vi "Force Analysis iso.vi"(1 "Dynamic Data Type 2":dynamicdata(waveform)) -> (0 "Dynamic Data Type":dynamicdata(waveform))   [LabVIEW 2016]
uses:
  <vilib>/express/express shared/transition.llb/Dynamic To Waveform Array.vi
  <vilib>/express/express arith-compare/Formula/Block/exnFormulaBlock how many pts in the wave.vi
  <vilib>/express/express shared/ex_Modify Signal Name.vi
  <vilib>/express/express shared/transition.llb/Waveform Array To Dynamic.vi
  <vilib>/express/express arith-compare/Formula/XNode/ExpressFormulaBlockNode.xnode
panel:
  in  "Tab Control":enum32{"Trial A"}(tab)
  out "RFD (PF)":dbl
  out "T to PF (ms)":dbl
  out "Min. Force":dbl
  out "Mean Force":dbl
  out "Impulse-250":dbl
  out "Impulse-200":dbl
  out "Impulse-150":dbl
  out "Impulse-100":dbl
  out "Impulse-PF":dbl
  out "F200":dbl
  out "RFD (250ms)":dbl
  out "RFD (150ms)":dbl
  out "RFD (100ms)":dbl
  out "F250":dbl
  out "F150":dbl
  out "F100":dbl
  out "RFD (200ms)":dbl
  out "PF":dbl
  out "Trial A":dynamicdata(graph) caption="Filtered Signal"
  out "PRFD (5ms)":dbl
  out "PRFD (10ms)":dbl
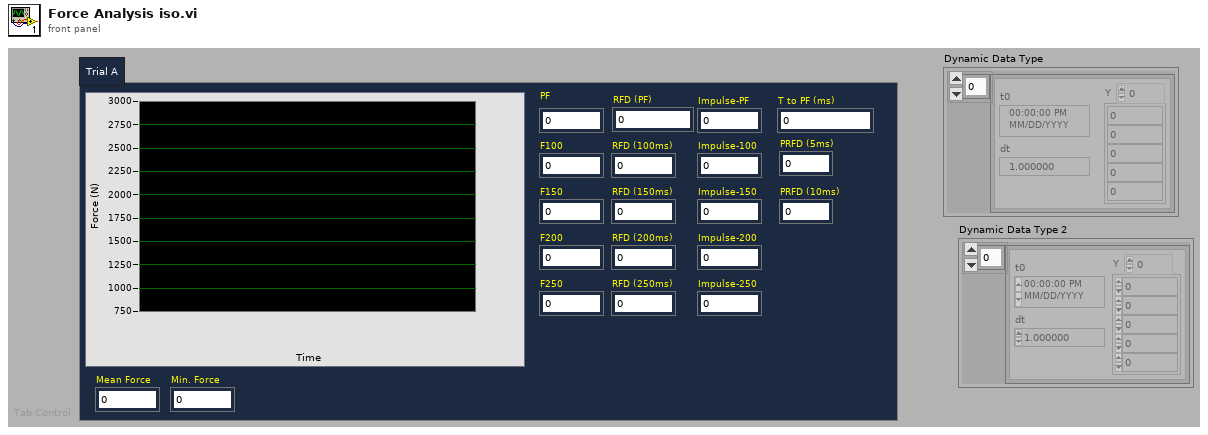
[diagram p1: front panel]
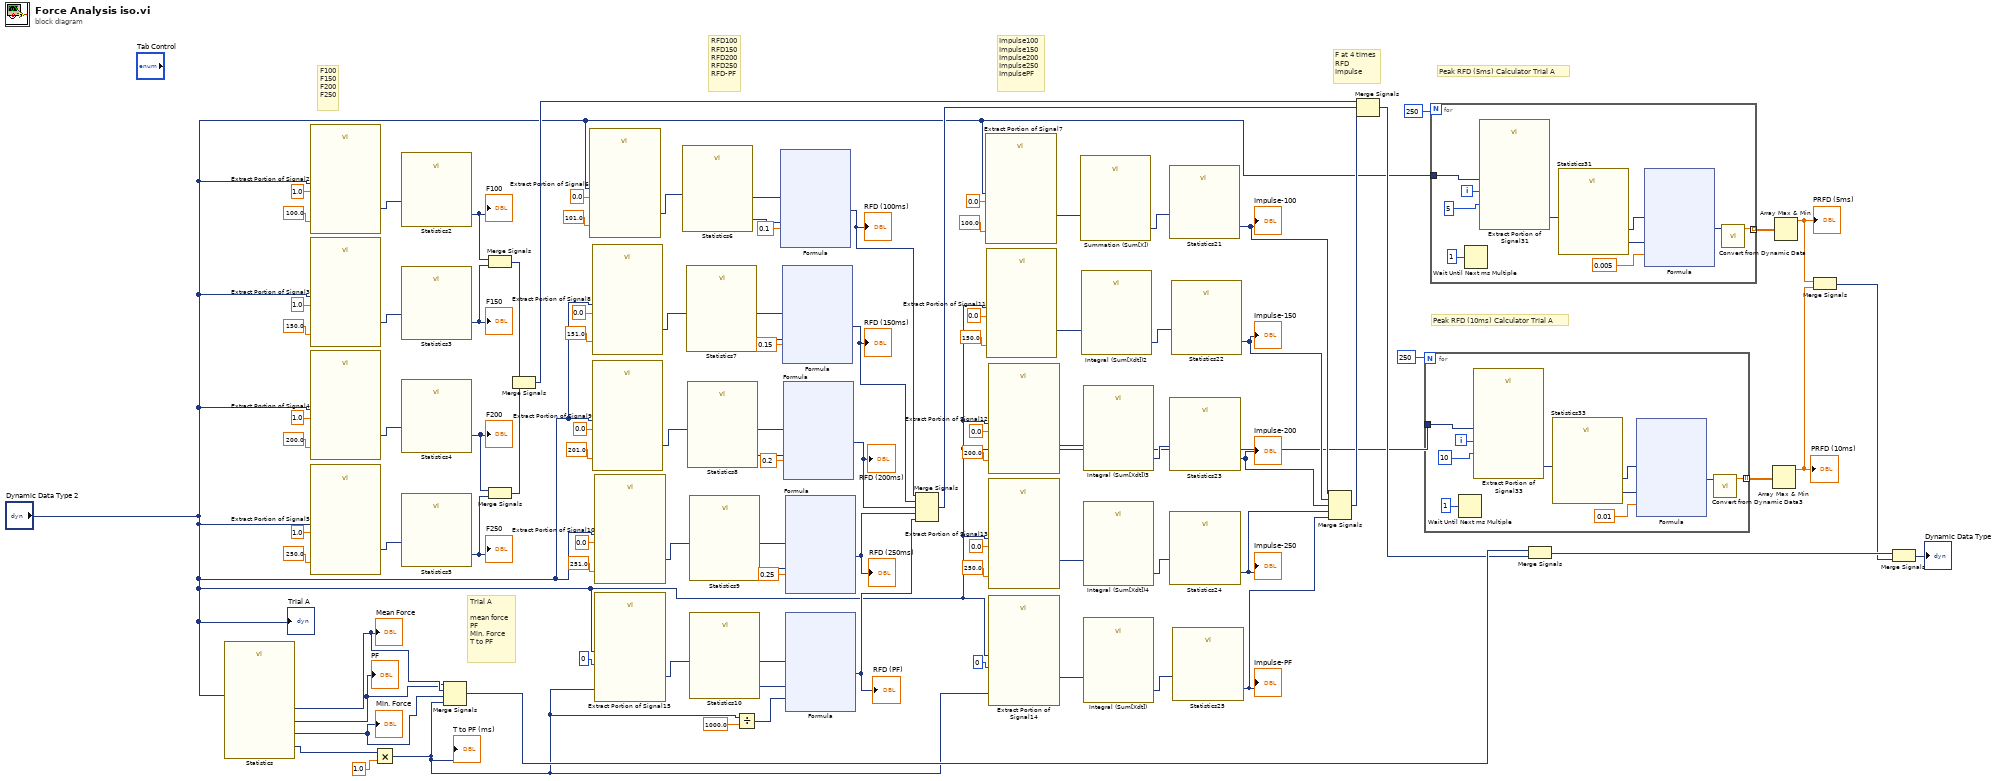
[diagram p0: block diagram]
diagram:
  # "Peak RFD (10ms) Calculator Trial A"
  # "Peak RFD (5ms) Calculator Trial A"
  # "F at 4 times\nRFD\nImpulse"
  # "Impulse100\nImpulse150\nImpulse200\nImpulse250\nImpulsePF"
  # "RFD100\nRFD150\nRFD200\nRFD250\nRFD-PF"
  # "Trial A\n\nmean force\nPF\nMin. Force\nT to PF"
  # "F100\nF150\nF200\nF250"
  n1 = call "Statistics"("Signals"="Dynamic Data Type 2") -> ("Index of Max"=w3:dynamicdata, "Arithmetic Mean"=w2:dynamicdata, "Minimum"=w16:dynamicdata, "Maximum"=w1:dynamicdata)  [unwired: 2 in, 21 out]
  "PF" <- w1
  "Mean Force" <- w2
  "Min. Force" <- w16
  n2 = call "Extract Portion of Signal2"("Samples"=100.0 ("y"), "Begin Sample"=1.0 ("y"), "Signals"="Dynamic Data Type 2") -> ("Section"=w95:dynamicdata)  [unwired: 1 in, 7 out]
  n3 = call "Extract Portion of Signal3"("Samples"=150.0 ("y"), "Begin Sample"=1.0 ("y"), "Signals"="Dynamic Data Type 2") -> ("Section"=w92:dynamicdata)  [unwired: 1 in, 7 out]
  n4 = call "Extract Portion of Signal4"("Samples"=200.0 ("y"), "Begin Sample"=1.0 ("y"), "Signals"="Dynamic Data Type 2") -> ("Section"=w89:dynamicdata)  [unwired: 1 in, 7 out]
  n5 = call "Extract Portion of Signal5"("Samples"=250.0 ("y"), "Begin Sample"=1.0 ("y"), "Signals"="Dynamic Data Type 2") -> ("Section"=w86:dynamicdata)  [unwired: 1 in, 7 out]
  n6 = Multiply(x=w3, y=1.0) -> (x*y=w5:dynamicdata)
  "T to PF (ms)" <- w5
  n7 = call "Statistics2"("Signals"=w95) -> ("Last Value"=w37:dynamicdata)  [unwired: 1 in, 25 out]
  "F100" <- w37
  n8 = call "Statistics3"("Signals"=w92) -> ("Last Value"=w38:dynamicdata)  [unwired: 1 in, 25 out]
  "F150" <- w38
  n9 = call "Statistics4"("Signals"=w89) -> ("Last Value"=w40:dynamicdata)  [unwired: 1 in, 25 out]
  "F200" <- w40
  n10 = call "Statistics5"("Signals"=w86) -> ("Last Value"=w39:dynamicdata)  [unwired: 1 in, 25 out]
  "F250" <- w39
  n11 = Merge Signals(w1, w2, w16, w5) -> (w15:dynamicdata)
  n12 = Merge Signals(w37, w38) -> (w36:dynamicdata)
  n13 = Merge Signals(w40, w39) -> (w35:dynamicdata)
  n14 = Merge Signals(w36, w35) -> (w17:dynamicdata)
  n15 = call "Extract Portion of Signal6"("Samples"=101.0 ("y"), "Begin Sample"=0.0 ("y"), "Signals"="Dynamic Data Type 2") -> ("Section"=w81:dynamicdata)  [unwired: 1 in, 7 out]
  n16 = call "Extract Portion of Signal8"("Samples"=151.0 ("y"), "Begin Sample"=0.0 ("y"), "Signals"="Dynamic Data Type 2") -> ("Section"=w72:dynamicdata)  [unwired: 1 in, 7 out]
  n17 = call "Extract Portion of Signal9"("Samples"=201.0 ("y"), "Begin Sample"=0.0 ("y"), "Signals"="Dynamic Data Type 2") -> ("Section"=w66:dynamicdata)  [unwired: 1 in, 7 out]
  n18 = call "Extract Portion of Signal10"("Samples"=251.0 ("y"), "Begin Sample"=0.0 ("y"), "Signals"="Dynamic Data Type 2") -> ("Section"=w60:dynamicdata)  [unwired: 1 in, 7 out]
  n19 = call "Extract Portion of Signal15"("Samples"=w5, "Begin Sample"=0, "Signals"="Dynamic Data Type 2") -> ("Section"=w45:dynamicdata)  [unwired: 1 in, 7 out]
  n20 = call "Statistics6"("Signals"=w81) -> ("Last Value"=w82:dynamicdata, "First Value"=w83:dynamicdata)  [unwired: 1 in, 24 out]
  n21 = call "Statistics7"("Signals"=w72) -> ("Last Value"=w73:dynamicdata, "First Value"=w74:dynamicdata)  [unwired: 1 in, 24 out]
  n22 = call "Statistics8"("Signals"=w66) -> ("Last Value"=w67:dynamicdata, "First Value"=w68:dynamicdata)  [unwired: 1 in, 24 out]
  n23 = call "Statistics9"("Signals"=w60) -> ("Last Value"=w61:dynamicdata, "First Value"=w62:dynamicdata)  [unwired: 1 in, 24 out]
  n24 = call "Statistics10"("Signals"=w45) -> ("Last Value"=w46:dynamicdata, "First Value"=w47:dynamicdata)  [unwired: 1 in, 24 out]
  n25 = Divide(x=w5, y=1000.0) -> (x/y=w43:dynamicdata)
  n26 = xnode "Formula"("first value"=w83, "last value"=w82, "X3"=0.1) -> ("Result"=w34:dynamicdata)  [unwired: 1 in, 1 out]
  "RFD (100ms)" <- w34
  n27 = xnode "Formula"("first value"=w74, "last value"=w73, "X3"=0.15) -> ("Result"=w33:dynamicdata)  [unwired: 1 in, 1 out]
  "RFD (150ms)" <- w33
  n28 = xnode "Formula"("first value"=w68, "last value"=w67, "X3"=0.2) -> ("Result"=w32:dynamicdata)  [unwired: 1 in, 1 out]
  "RFD (200ms)" <- w32
  n29 = xnode "Formula"("first value"=w62, "last value"=w61, "X3"=0.25) -> ("Result"=w31:dynamicdata)  [unwired: 1 in, 1 out]
  "RFD (250ms)" <- w31
  n30 = xnode "Formula"("first value"=w47, "last value"=w46, "X3"=w43) -> ("Result"=w30:dynamicdata)  [unwired: 1 in, 1 out]
  "RFD (PF)" <- w30
  n31 = Merge Signals(w34, w33, w32, w31, w30) -> (w18:dynamicdata)
  n32 = call "Extract Portion of Signal7"("Samples"=100.0 ("y"), "Begin Sample"=0.0 ("y"), "Signals"="Dynamic Data Type 2") -> ("Section"=w78:dynamicdata)  [unwired: 1 in, 7 out]
  n33 = call "Extract Portion of Signal11"("Samples"=150.0 ("y"), "Begin Sample"=0.0 ("y"), "Signals"="Dynamic Data Type 2") -> ("Section"=w56:dynamicdata)  [unwired: 1 in, 7 out]
  n34 = call "Extract Portion of Signal12"("Samples"=200.0 ("y"), "Begin Sample"=0.0 ("y"), "Signals"="Dynamic Data Type 2") -> ("Section"=w53:dynamicdata)  [unwired: 1 in, 7 out]
  n35 = call "Extract Portion of Signal13"("Samples"=250.0 ("y"), "Begin Sample"=0.0 ("y"), "Signals"="Dynamic Data Type 2") -> ("Section"=w50:dynamicdata)  [unwired: 1 in, 7 out]
  n36 = call "Extract Portion of Signal14"("Samples"=w5, "Begin Sample"=0, "Signals"="Dynamic Data Type 2") -> ("Section"=w48:dynamicdata)  [unwired: 1 in, 7 out]
  n37 = call "Summation (Sum[X])"("Signals"=w78) -> ("Result"=w29:dynamicdata)  [unwired: 1 in, 5 out]
  n38 = call "Integral (Sum[Xdt])2"("Signals"=w56) -> ("Result"=w28:dynamicdata)  [unwired: 1 in, 5 out]
  n39 = call "Integral (Sum[Xdt])3"("Signals"=w53) -> ("Result"=w27:dynamicdata)  [unwired: 1 in, 5 out]
  n40 = call "Integral (Sum[Xdt])4"("Signals"=w50) -> ("Result"=w26:dynamicdata)  [unwired: 1 in, 5 out]
  n41 = call "Integral (Sum[Xdt])"("Signals"=w48) -> ("Result"=w25:dynamicdata)  [unwired: 1 in, 5 out]
  n42 = call "Statistics21"("Signals"=w29) -> ("Last Value"=w24:dynamicdata)  [unwired: 1 in, 25 out]
  "Impulse-100" <- w24
  n43 = call "Statistics23"("Signals"=w27) -> ("Last Value"=w22:dynamicdata)  [unwired: 1 in, 25 out]
  "Impulse-200" <- w22
  n44 = call "Statistics24"("Signals"=w26) -> ("Last Value"=w21:dynamicdata)  [unwired: 1 in, 25 out]
  "Impulse-250" <- w21
  n45 = call "Statistics22"("Signals"=w28) -> ("Last Value"=w23:dynamicdata)  [unwired: 1 in, 25 out]
  "Impulse-150" <- w23
  n46 = call "Statistics25"("Signals"=w25) -> ("Last Value"=w20:dynamicdata)  [unwired: 1 in, 25 out]
  "Impulse-PF" <- w20
  n47 = Merge Signals(w24, w23, w22, w21, w20) -> (w19:dynamicdata)
  n48 = Merge Signals(w17, w18, w19) -> (w14:dynamicdata)
  n49 = for {
    N: 250 -> [_]
    tunnel: [w100] -> w10 mode=indexing
    tunnel: "Dynamic Data Type 2" -> [w99]
    i -> [w103]
    n50 = Wait Until Next ms Multiple(millisecond multiple=1) -> ()  [unwired: 1 out]
    n51 = call "Extract Portion of Signal33"("Samples"=10, "Begin Sample"=w103, "Signals"=w99) -> ("Section"=w107:dynamicdata)  [unwired: 1 in, 7 out]
    n52 = call "Statistics33"("Signals"=w107) -> ("Last Value"=w106:dynamicdata, "First Value"=w105:dynamicdata)  [unwired: 1 in, 24 out]
    n53 = xnode "Formula"("first value"=w105, "last value"=w106, "X3"=0.01) -> ("Result"=w101:dynamicdata)  [unwired: 1 in, 1 out]
    n54 = call "Convert from Dynamic Data3"("Dynamic Data Type"=w101) -> ("Array"=w100:dbl[])  [unwired: 3 out]
  }
  n55 = for {
    N: 250 -> [_]
    tunnel: [w249] -> w12 mode=indexing
    tunnel: "Dynamic Data Type 2" -> [w248]
    i -> [w252]
    n56 = Wait Until Next ms Multiple(millisecond multiple=1) -> ()  [unwired: 1 out]
    n57 = call "Extract Portion of Signal31"("Samples"=5, "Begin Sample"=w252, "Signals"=w248) -> ("Section"=w256:dynamicdata)  [unwired: 1 in, 7 out]
    n58 = call "Statistics31"("Signals"=w256) -> ("Last Value"=w255:dynamicdata, "First Value"=w254:dynamicdata)  [unwired: 1 in, 24 out]
    n59 = xnode "Formula"("first value"=w254, "last value"=w255, "X3"=0.005) -> ("Result"=w250:dynamicdata)  [unwired: 1 in, 1 out]
    n60 = call "Convert from Dynamic Data"("Dynamic Data Type"=w250) -> ("Array"=w249:dbl[])  [unwired: 3 out]
  }
  n61 = Merge Signals(w15, w14) -> (w9:dynamicdata)
  n62 = Array Max & Min(array=w10) -> (max value=w7:dbl)  [unwired: 3 out]
  "PRFD (10ms)" <- w7
  n63 = Array Max & Min(array=w12) -> (max value=w8:dbl)  [unwired: 3 out]
  "PRFD (5ms)" <- w8
  n64 = Merge Signals(w8, w7) -> (w6:dynamicdata)
  n65 = Merge Signals(w9, w6) -> (→"Dynamic Data Type":dynamicdata)
  "Trial A" <- "Dynamic Data Type 2"
